vi "Digital Output - N Channel - 1 Sample.vi"() -> ()   [LabVIEW 2019]
uses:
  <vilib>/myRIO/Common/Instrument Driver Framework/ELVIS III v1.0/DIO/vis/ELVIS III v1.0 Close DIO.vi
  <vilib>/myRIO/Common/Instrument Driver Framework/myRIO v1.0/UART/vis/myRIO v1.0 Close UART.vi
  <vilib>/myRIO/Common/Instrument Driver Framework/ELVIS III v1.0/DIO/vis/ELVIS III v1.0 Unreserve DIO.vi
  <vilib>/myRIO/Common/Instrument Driver Framework/ELVIS III v1.0/DIO/vis/ELVIS III v1.0 Build MUX Configuration DIO.vi
  <vilib>/myRIO/Common/Instrument Driver Framework/ELVIS III v1.0/Resource Manager/vis/ELVIS III v1.0 Create Configuration List.vi
  <vilib>/Utility/error.llb/Error Cluster From Error Code.vi
  <vilib>/myRIO/Common/Instrument Driver Framework/ELVIS III v1.0/DIO/vis/ELVIS III v1.0 Write DIO.vi
  <vilib>/myRIO/Common/Instrument Driver Framework/ELVIS III v1.0/DIO/vis/ELVIS III v1.0 Shutdown DIO.vi
  <vilib>/myRIO/Common/Instrument Driver Framework/ELVIS III v1.0/Resource Manager/vis/ELVIS III v1.0 Configure IO.vi
  <vilib>/myRIO/Common/Instrument Driver Framework/ELVIS III v1.0/Resource Manager/vis/ELVIS III v1.0 Unreserve Channel List.vi
  <vilib>/myRIO/Common/Instrument Driver Framework/myRIO v1.0/myRIO v1.0 Close.vi
  <vilib>/myRIO/Common/Instrument Driver Framework/Utilities/vis/FPGA Ref Manager.vi
  <vilib>/myRIO/Common/Instrument Driver Framework/ELVIS III v1.0/ELVIS III v1.0 Reset FPGA.vi
  <vilib>/myRIO/Common/Instrument Driver Framework/myRIO v1.0/IRQ/vis/myRIO v1.0 IRQ Info FGV.vi
  <vilib>/myRIO/Common/Instrument Driver Framework/myRIO v1.0/IRQ/vis/myRIO v1.0 Timer IRQ Info FGV.vi
  <vilib>/myRIO/Common/Instrument Driver Framework/myRIO v1.0/IRQ/vis/myRIO v1.0 ISR Agent.vi
  <vilib>/myRIO/Instrument Drivers/Utilities/vis/Reset Index.vi
  <vilib>/myRIO/Common/Instrument Driver Framework/myRIO v1.0/Resource Manager/vis/myRIO v1.0 Block Write Resource Manager.vi
  <vilib>/myRIO/Instrument Drivers/Onboard IO/DIO/DIO.lvlib
  <vilib>/myRIO/Instrument Drivers/Utilities/Utilities.lvlib
panel:
  in  "A/DIO1":bool
  in  "Stop":bool
  in  "A/DIO0":bool
  # "ELVIS III Control IO"
  # "数字输出N通道"
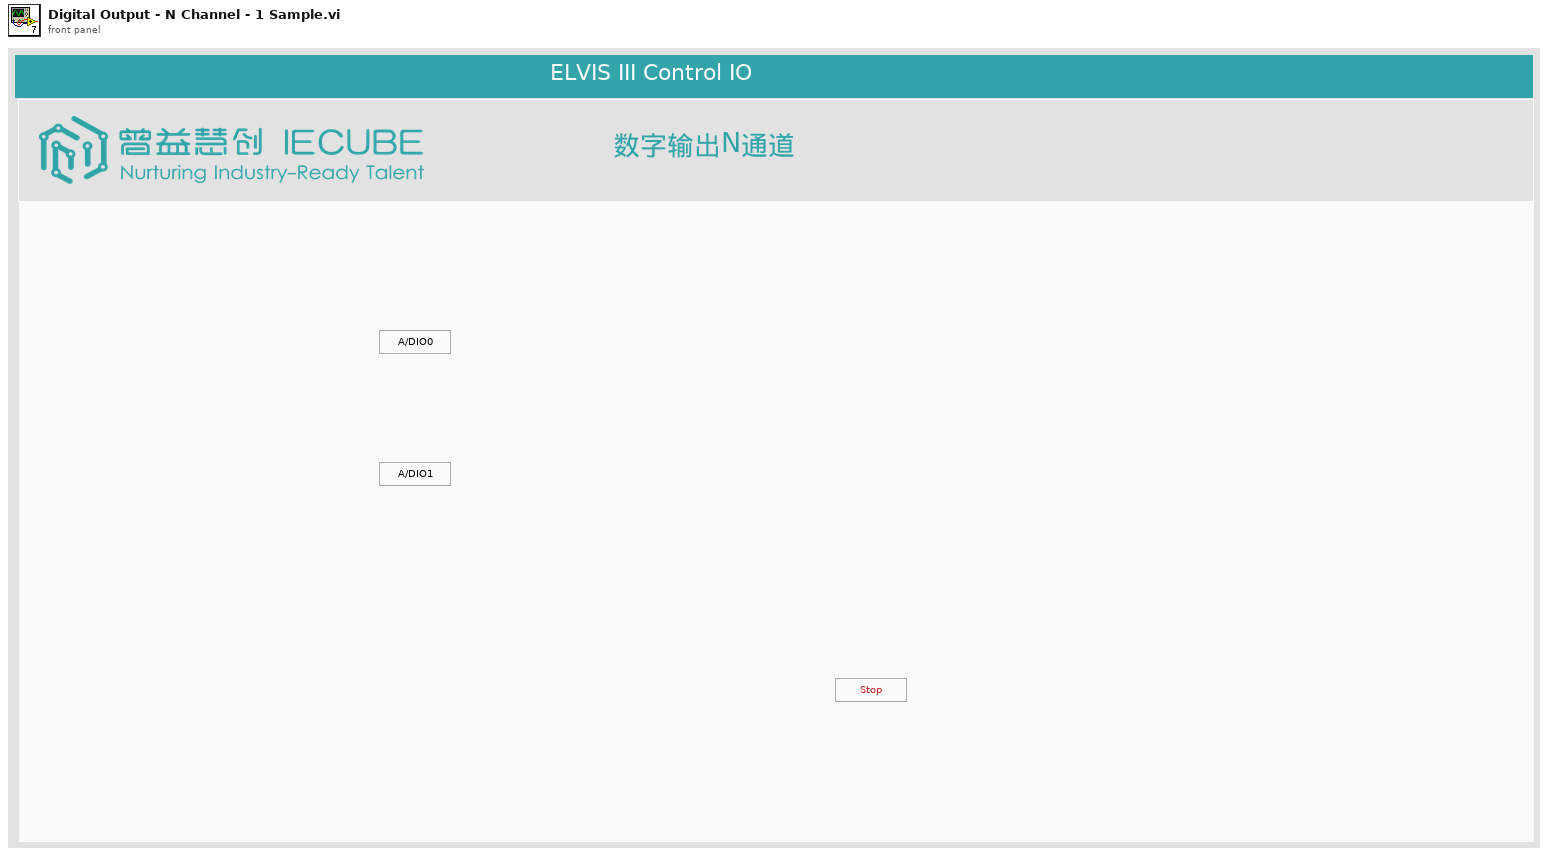
[diagram p1: front panel]
types:
  T1 = typedef "DIO.lvlib/DIO Reference.ctl" = cluster{"myRIO Reference":T2, "DIO Channels List":T6}
  T2 = typedef "myRIO Generic Hardware Reference.ctl" = cluster{"myRIO Model":T3, "myRIO Hardware Reference":T4}
  T3 = typedef "Hardware Version Enum.ctl" = enum16{"Unknown", "myRIO-1900", "myRIO-1950", "roboRIO", "NI ELVIS RIO CM", "ELVIS III"}
  T4 = typedef "myRIO v1.0 Reference.ctl" = cluster{"Generic FPGA Reference":T5, "Allow multiple opens":bool}
  T5 = typedef "Generic FPGA Reference.ctl" = refnum<k20>
  T6 = typedef "DIO Channels List.ctl" = T7[]
  T7 = typedef "DIO Channels Enum.ctl" = enum16{"Not Connected", "C/DIO0", "C/DIO1", "C/DIO2", "C/DIO3", "C/DIO4", "C/DIO5", "C/DIO6", "C/DIO7", "A/DIO0", "A/DIO1", "A/DIO2", "A/DIO3", "A/DIO4", "A/DIO5", "A/DIO6", "A/DIO7", "A/DIO8", "A/DIO9", "A/DIO10", "A/DIO11", "A/DIO12", "A/DIO13", "A/DIO14", "A/DIO15", "A/DIO16", "A/DIO17", "A/DIO18", "A/DIO19", "B/DIO0", "B/DIO1", "B/DIO2", "B/DIO3", "B/DIO4", "B/DIO5", "B/DIO6", "B/DIO7", "B/DIO8", "B/DIO9", "B/DIO10", "B/DIO11", "B/DIO12", "B/DIO13", "B/DIO14", "B/DIO15", "B/DIO16", "B/DIO17", "B/DIO18", "B/DIO19", "LED0", "LED1", "LED2", "LED3", "Button0", "DIO/DIO0", "DIO/DIO1", "DIO/DIO2", "DIO/DIO3", "DIO/DIO4", "DIO/DIO5", "DIO/DIO6", "DIO/DIO7", "DIO/DIO8", "DIO/DIO9", "SPI/CS0", "SPI/CS1", "SPI/CS2", "SPI/CS3", "LED RADIO (Green)", "LED RADIO (Red)", "LED COMM (Green)", "LED COMM (Red)", "LED MODE (Green)", "LED MODE (Red)"}
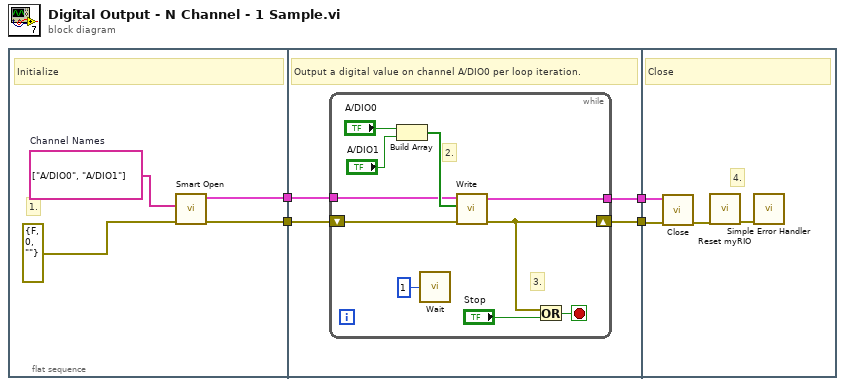
[diagram p0: block diagram]
diagram:
  n1 = flat-sequence {
    tunnel: [w6] -> w4
    tunnel: [w5] -> w3
    tunnel: [w12] -> w2
    tunnel: w4 -> [w11]
    tunnel: w3 -> [w10]
    tunnel: [w9] -> w1
    tunnel: w2 -> [w25]
    tunnel: w1 -> [w23]
    frame #0 {
      w8 = tag[] ["A/DIO0", "A/DIO1"]  # Channel Names
      # "1."
      # "Initialize"
      n2 = call <vilib>:"Smart Open.vi"("error in (no error)"=errorcluster {"status"=FALSE, "code"=0, "source"=""} ("Error In"), "Channel Names"=w8) -> ("error out"=w6:errorcluster, "DIO Ref Out"=w5:T1)  [unwired: 8 in]
    }
    frame #1 {
      # "Output a digital value on channel A/DIO0 per loop iteration."
      n3 = while {
        shift-right: [w16] -> w12
        shift-left: w11 -> [w17]
        tunnel: w10 -> [w15]
        tunnel: [w14] -> w9
        stop <- w22 stop-if-true
        # "3."
        # "2."
        n4 = Build Array("A/DIO0", "A/DIO1") -> (w19:bool[])
        n5 = call "Wait"("Count(mSec)"=u32 1) -> ()  [unwired: 1 out]
        n6 = call <vilib>:"Write.vi"("error in (no error)"=w17, "Values"=w19, "DIO Ref In"=w15) -> ("error out"=w16:errorcluster, "DIO Ref Out"=w14:T1)  [unwired: 6 in]
        n7 = Or(x=w16, y="Stop") -> (x .or. y?=w22:bool)
      }
    }
    frame #2 {
      # "4."
      # "Close"
      n8 = call <vilib>:"Close.vi"("error in (no error)"=w25, "DIO Ref In"=w23) -> ("error out"=w24:errorcluster)  [unwired: 9 in]
      n9 = call <vilib>:"Reset myRIO.vi"("error in (no error)"=w24) -> ("error out"=w26:errorcluster)  [unwired: 10 in]
      n10 = call <vilib>:"Simple Error Handler.vi"("error in (no error)"=w26) -> ()  [unwired: 4 in, 5 out]
    }
  }
